vi "DPIDs.Export.vi"(8 "error in (no error)":errorcluster, 11 "Section Ref in":T1 format="%.0x") -> (0 "error out":errorcluster, 2 "DPIDs":T2, 3 "Section Ref out":T1 format="%.0x")   [LabVIEW 2015, in "Diagnostics Addon System Explorer.lvlib"]
uses:
  Diagnostics Addon System Explorer.lvlib
  <vilib>/NI Veristand/Custom Device API/Custom Device Item Ref.ctl
  Types/DPIDs.Export.ctl
  Types/DPID.Export.ctl
  Shared/Types/DPID.ctl
  Shared/Types/DPID.Rate.ctl
  Types/FG.Action.ctl
  ID.FG.vi
  <vilib>/NI Veristand/Custom Device API/NI VeriStand - Get Item Property.vi
  <vilib>/NI Veristand/Custom Device API/Get Item Property (U32 Array).vi
  <vilib>/NI Veristand/Custom Device API/Get Item Property (U32).vi
  <vilib>/NI Veristand/Custom Device API/NI VeriStand - Set Item Property.vi
  <vilib>/NI Veristand/Custom Device API/Set Item Property (U32).vi
  Shared/SubVIs/Constants.vi
  <vilib>/NI Veristand/Custom Device API/Set Item Property (U32 Array).vi
  <vilib>/NI Veristand/Custom Device Tools/Custom Device Utility Library/NI VeriStand - Search for Item by GUID.vi
  <vilib>/NI Veristand/Custom Device Tools/Custom Device Utility Library/Custom Device Utility Library.lvlib
  Shared/Diagnostics Addon Shared.lvlib
  <vilib>/NI Veristand/Custom Device API/Custom Device API.lvlib
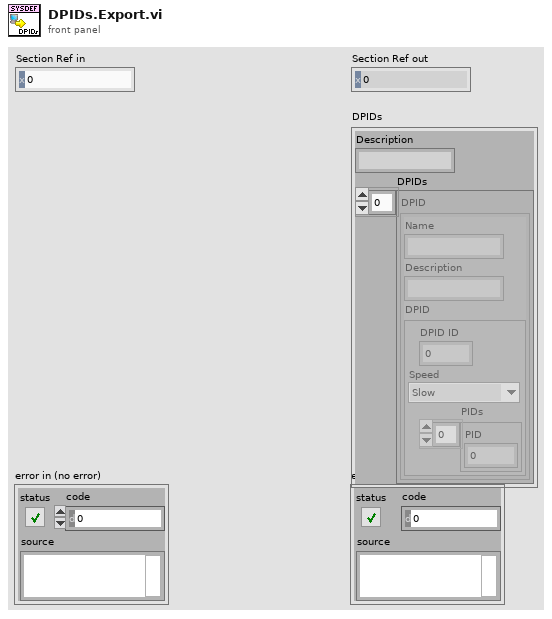
[diagram p1: front panel]
types:
  T1 = typedef "Custom Device API.lvlib/Custom Device Item Ref.ctl" = u64
  T2 = typedef "Diagnostics Addon System Explorer.lvlib/DPIDs.Export.ctl" = cluster{"Description":string, "DPIDs":T3[]}
  T3 = typedef "Diagnostics Addon System Explorer.lvlib/DPID.Export.ctl" = cluster{"Name":string, "Description":string, "DPID":T4}
  T4 = typedef "Diagnostics Addon Shared.lvlib/DPID.ctl" = cluster{"DPID ID":u8, "Speed":T5, "PIDs":u16[]}
  T5 = typedef "Diagnostics Addon Shared.lvlib/DPID.Rate.ctl" = enum16{"Slow", "Medium", "Fast"}
  T6 = typedef "Diagnostics Addon System Explorer.lvlib/FG.Action.ctl" = enum16{"Get", "Set"}
  T7 = typedef "Custom Device API.lvlib/Custom Device Item Info.ctl" = cluster{"Name":string, "Is Channel":bool, "GUID":string, "Is Waveform":bool}
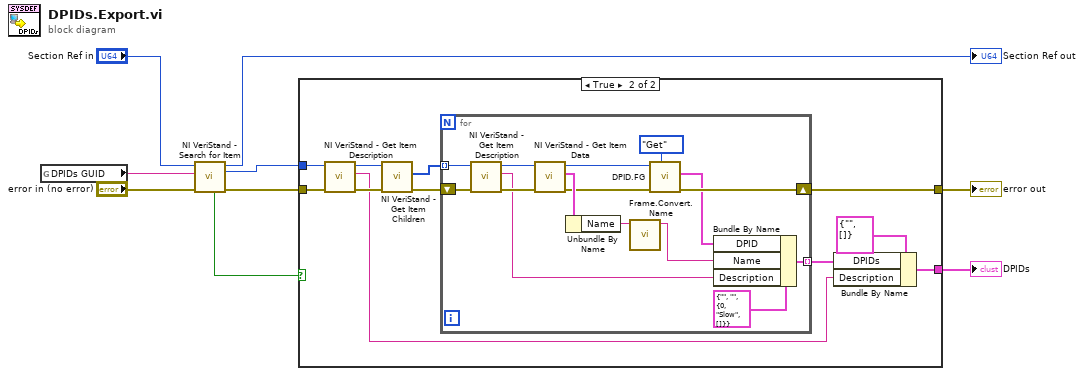
[diagram p0: block diagram]
diagram:
  n1 = global read "Constants.vi" "DPIDs GUID"() -> (w1:string)
  n2 = call-poly <vilib>:"NI VeriStand - Search for Item.vi"("error in"="error in (no error)", "Item GUID"=w1, "Section Ref in"="Section Ref in") -> ("error out"=w9:errorcluster, "Item Ref"=w8:T1, "Section Ref out"=→"Section Ref out":T1, "Found"=w7:bool)  [unwired: 5 in]
  n3 = case shown="True" w7 {
    tunnel: w8 -> [_ w16]
    tunnel: w9 -> [w10 w17]
    tunnel: [w10 w20] -> w5
    tunnel: [_ w11] -> w4
    frame False {
    }
    frame True {
      n4 = call <vilib>:"NI VeriStand - Get Item Description.vi"("error in (no error)"=w17, "Item Ref in"=w16) -> ("error out"=w14:errorcluster, "Description"=w13:string, "Item Ref out"=w15:T1)  [unwired: 7 out]
      n5 = call <vilib>:"NI VeriStand - Get Item Children.vi"("error in (no error)"=w14, "Item Ref in"=w15) -> ("error out"=w21:errorcluster, "Child Refs"=w19:T1[])  [unwired: 6 in, 2 out]
      n6 = for {
        tunnel: w19 -> [w32] mode=indexing
        tunnel: [w30] -> w12 mode=indexing
        shift-right: [w27] -> w20
        shift-left: w21 -> [w33]
        n7 = call <vilib>:"NI VeriStand - Get Item Description.vi"("error in (no error)"=w33, "Item Ref in"=w32) -> ("error out"=w35:errorcluster, "Description"=w31:string, "Item Ref out"=w34:T1)  [unwired: 7 out]
        n8 = call <vilib>:"NI VeriStand - Get Item Data.vi"("error in (no error)"=w35, "Item Ref in"=w34) -> ("error out"=w29:errorcluster, "Item Info"=w36:T7, "Item Ref out"=w28:T1)  [unwired: 7 out]
        n9 = Unbundle By Name(w36) -> ("Name"=w23:string)
        n10 = call "Frame.Convert.Name.vi"("VS Frame Name"=w23) -> ("Frame Name"=w22:string)  [unwired: 9 in, 1 out]
        n11 = call "DPID.FG.vi"("Action"=FG.Action."Get", "error in (no error)"=w29, "Device Item Ref in"=w28) -> ("error out"=w27:errorcluster, "DPID"=w24:T4)  [unwired: 6 in, 1 out]
        n12 = Bundle By Name(cluster=T3 {"Name"="", "Description"="", "DPID"={"DPID ID"=0, "Speed"=enum."Slow", "PIDs"=[]}} ("DPID"), "DPID"=w24, "Name"=w22, "Description"=w31) -> (w30:T3)
      }
      n13 = Bundle By Name(cluster=T2 {"Description"="", "DPIDs"=[]}, "DPIDs"=w12, "Description"=w13) -> (w11:T2)
    }
  }
  "error out" <- w5
  "DPIDs" <- w4
